vi "SM-UI.vi"() -> ()   [LabVIEW 2024]
uses:
  TypeDefs/SM-States.ctl
panel:
  out "Komunikaty":string
  out "HistoryGraph":cluster{"X":dbl, "Y":dbl}[](graph)
  out "unit":string
  out "timestamp":u64
  out "value":dbl
  out "sensor":string
  out "device_id":string
  in  "History":bool
  in  "Latest":bool
  in  "Limit":dbl
  in  "Sensors":u16(ring) items=["temp", "hum", "pressure"]
  in  "Device":u16(ring) items=["esp32-abcd01", "esp32-abcd03", "esp32-abcd02"]
  in  "Refresh Interval":i32
  in  "Auto Refresh":bool
  in  "Refresh":bool
  in  "Test API":bool
  out "StatusAPI":string
  in  "API-URL":string
  in  "stop":bool
  # "Rozproszone Systemy Pomiarowe - Dasboard LabVIEW"
  # "REST API URL:"
  # "Status API:"
  # "Konfiguracja i filtry"
  # "Device"
  # "Sensor"
  # "Limit"
  # "Latest measurement"
  # "Device ID"
  # "Sensor"
  # "Value"
  # "Unit"
  # "TimeStamp"
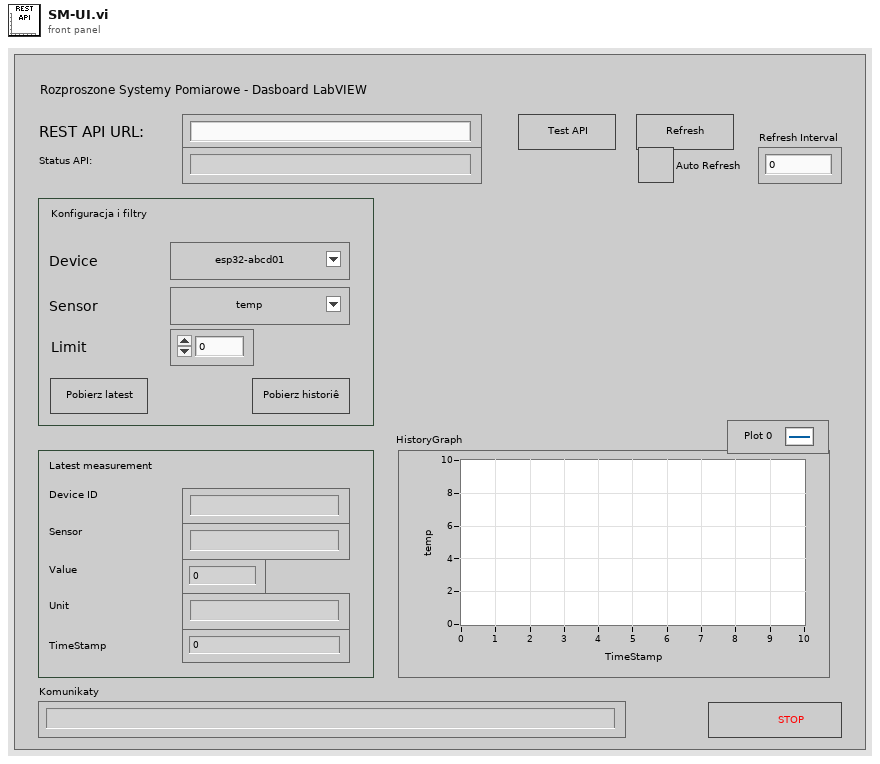
[diagram p1: front panel]
types:
  T1 = typedef "SM-States.ctl" = enum16{"Init", "Stop", "TestAPI", "Refresh", "Latest", "History", "LaadDevices", "DecWait"}
  T2 = typedef "MeasurementData.ctl" = cluster{"device_id":string, "sensor":string, "value":dbl, "unit":string, "group_id":string}
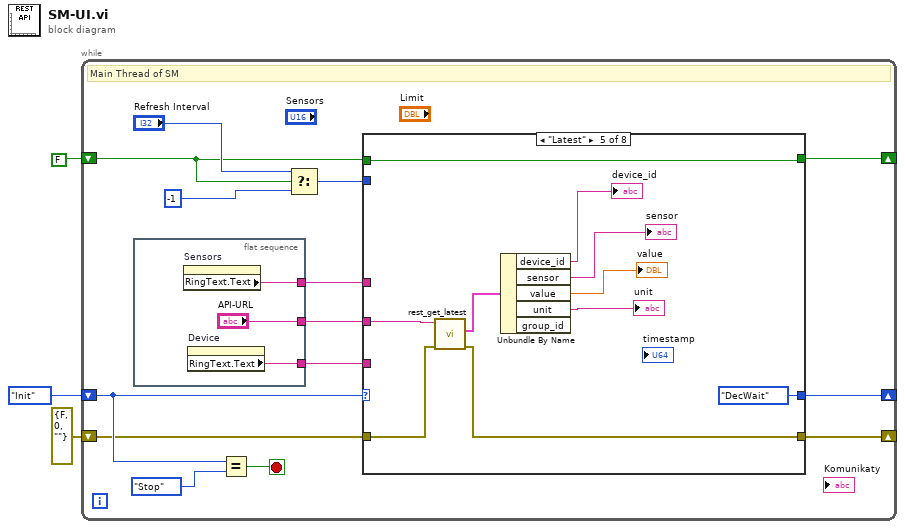
[diagram p0: block diagram]
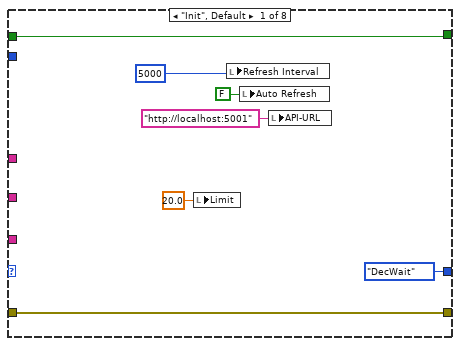
[diagram p2: hidden frame]
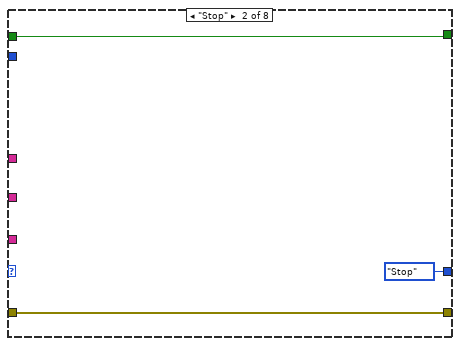
[diagram p3: hidden frame]
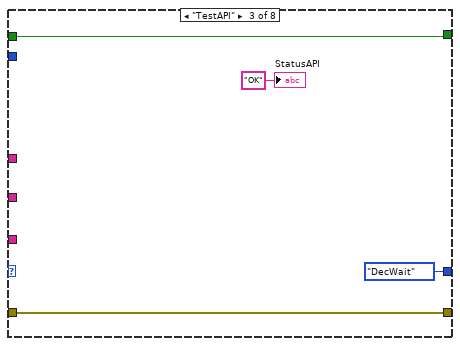
[diagram p4: hidden frame]
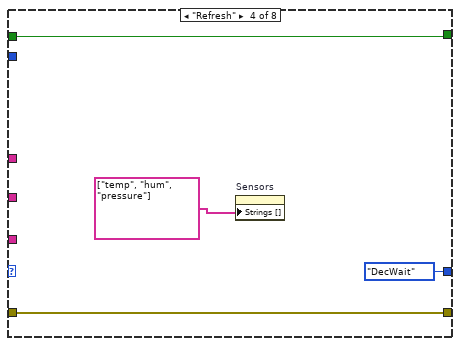
[diagram p5: hidden frame]
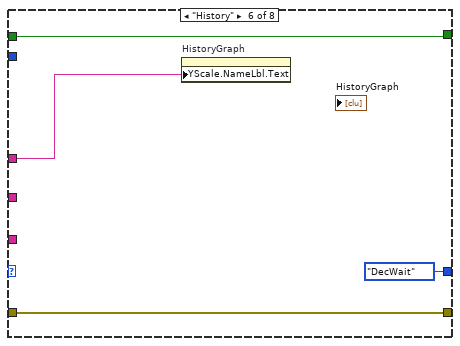
[diagram p6: hidden frame]
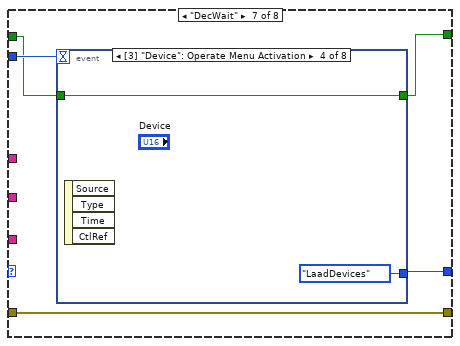
[diagram p7: hidden frame]
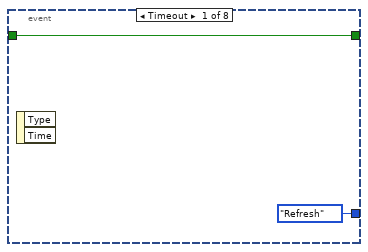
[diagram p8: hidden frame]
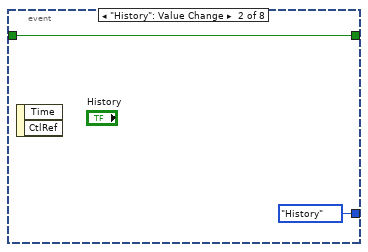
[diagram p9: hidden frame]
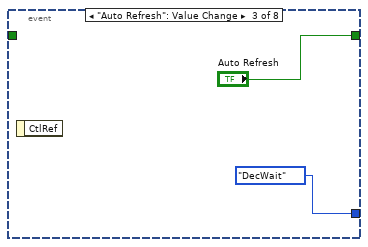
[diagram p10: hidden frame]
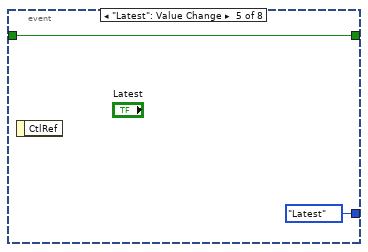
[diagram p11: hidden frame]
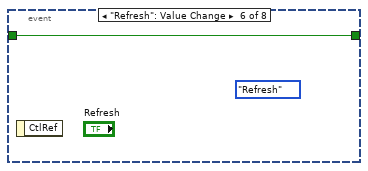
[diagram p12: hidden frame]
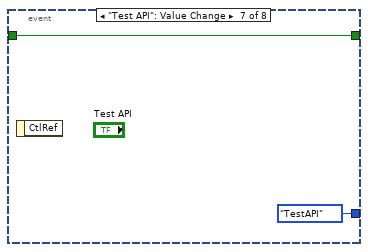
[diagram p13: hidden frame]
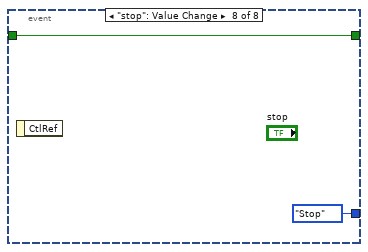
[diagram p14: hidden frame]
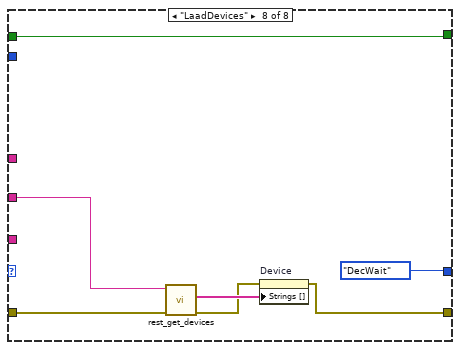
[diagram p15: hidden frame]
diagram:
  n1 = while {
    shift-right: [w7] -> _
    shift-left: SM-States."Init" ("CMD") -> [w10]
    shift-right: [w14] -> _
    shift-left: FALSE ("Auto Refresh") -> [w6]
    shift-right: [w5] -> _
    shift-left: errorcluster {"status"=FALSE, "code"=0, "source"=""} ("error out") -> [w4]
    stop <- w8 stop-if-true
    # "Main Thread of SM"
    n2 = flat-sequence {
      tunnel: [w20] -> w17
      tunnel: ["API-URL"] -> w16
      tunnel: [w18] -> w15
      frame #0 {
        n3 = property on="Sensors" class="Ring (strict)"() -> ("RingText.Text"=w20:string)  [unwired: 2 in, 2 out]
        n4 = property on="Device" class="Ring (strict)"() -> ("RingText.Text"=w18:string)  [unwired: 2 in, 2 out]
      }
    }
    n5 = Equal?(x=w10, y=SM-States."Stop") -> (x = y?=w8:bool)
    n6 = Select(t="Refresh Interval", s=w6, f=-1) -> (s? t:f=w11:i32)
    n7 = case shown="\"Latest\"" w10 {
      tunnel: w17 -> [_ _ _ _ _ w52 _ _]
      tunnel: w16 -> [_ _ _ _ w45 _ _ w77]
      tunnel: w15 -> [_ _ _ _ _ _ _ _]
      tunnel: [w23 w29 w32 w36 w47 w50 w57 w79] -> w14
      tunnel: w11 -> [_ _ _ _ _ _ w56 _]
      tunnel: [SM-States."DecWait" ("CMD") SM-States."Stop" ("CMD") SM-States."DecWait" ("CMD") SM-States."DecWait" ("CMD") SM-States."DecWait" ("CMD") SM-States."DecWait" ("CMD") w55 SM-States."DecWait" ("CMD")] -> w7
      tunnel: w6 -> [w23 w29 w32 w36 w47 w50 w54 w79]
      tunnel: [w21 w28 w31 w35 w39 w49 w53 w73] -> w5
      tunnel: w4 -> [w21 w28 w31 w35 w46 w49 w53 w76]
      frame "Init", Default {
        n8 = local write "Limit"(20.0 ("Limit")) -> ()
        n9 = local write "Refresh Interval"(5000 ("Refresh Interval")) -> ()
        n10 = local write "Auto Refresh"(FALSE ("Auto Refresh")) -> ()
        n11 = local write "API-URL"("http://localhost:5001" ("API-URL")) -> ()
      }
      frame "Stop" {
      }
      frame "TestAPI" {
        "StatusAPI" <- "OK" ("StatusAPI")
      }
      frame "Refresh" {
        n12 = property on="Sensors" class="Ring (strict)"("Strings []"=string[] ["temp", "hum", "pressure"]) -> ()  [unwired: 2 in, 2 out]
      }
      frame "Latest" {
        n13 = call "rest_get_latest.vi"("error in (no error)"=w46, "Base URL"=w45) -> ("error out"=w39:errorcluster, "value"=w44:T2)  [unwired: 8 in]
        n14 = Unbundle By Name(w44) -> ("device_id"=→"device_id":string, "sensor"=→"sensor":string, "value"=→"value":dbl, "unit"=→"unit":string)  [unwired: 1 out]
      }
      frame "History" {
        n15 = property on="HistoryGraph" class="XYGraph (strict)"("YScale.NameLbl.Text"=w52) -> ()  [unwired: 2 in, 2 out]
      }
      frame "DecWait" {
        n16 = event shown="[3] \"Device\": Operate Menu Activation" {
          selector: _ -> [_ _ _ _ _ _ _ _]
          dyn-events: _ -> [_ _ _ _ _ _ _ _]
          timeout: w56 -> [_ _ _ _ _ _ _ _]
          tunnel: [w58 w60 "Auto Refresh" w64 w67 w68 w69 w71] -> w57
          tunnel: [SM-States."Refresh" ("CMD") SM-States."History" ("CMD") SM-States."DecWait" ("CMD") SM-States."LaadDevices" ("CMD") SM-States."Latest" ("CMD") _ SM-States."TestAPI" ("CMD") SM-States."Stop" ("CMD")] -> w55
          tunnel: w54 -> [w58 w60 _ w64 w67 w68 w69 w71]
          event Timeout {
            n17 = event-data() -> ()  [unwired: 1 in, 2 out]
          }
          event "History": Value Change {
            n18 = event-data() -> ()  [unwired: 1 in, 2 out]
          }
          event "Auto Refresh": Value Change {
            n19 = event-data() -> ()  [unwired: 1 in, 1 out]
          }
          event "Device": Operate Menu Activation {
            n20 = event-data() -> ()  [unwired: 1 in, 4 out]
          }
          event "Latest": Value Change {
            n21 = event-data() -> ()  [unwired: 1 in, 1 out]
          }
          event "Refresh": Value Change {
            (unwired) SM-States."Refresh" ("CMD")
            n22 = event-data() -> ()  [unwired: 1 in, 1 out]
          }
          event "Test API": Value Change {
            n23 = event-data() -> ()  [unwired: 1 in, 1 out]
          }
          event "stop": Value Change {
            n24 = event-data() -> ()  [unwired: 1 in, 1 out]
          }
        }
      }
      frame "LaadDevices" {
        n25 = call "rest_get_devices.vi"("error in"=w76, "Base URL"=w77) -> ("error out"=w74:errorcluster, "DeviceArray"=w75:string[])  [unwired: 8 in]
        n26 = property on="Device" class="Ring (strict)"(error in=w74, "Strings []"=w75) -> (error out=w73:errorcluster)  [unwired: 1 in, 1 out]
      }
    }
  }
